vi "get_center.vi"(8 "error in (no error)":errorcluster, 11 "RoiGeneric in":refnum<class "RoiGeneric.lvclass">) -> (0 "error out":errorcluster, 2 "center":refnum<class "SpaceVector.lvclass">, 3 "RoiGeneric out":refnum<class "RoiGeneric.lvclass">)   [LabVIEW 2010, in "RoiGeneric.lvclass"]
uses:
  RoiGeneric.lvclass
  common/classes/SpaceVector/SpaceVector/SpaceVector.lvclass
  RoiGeneric.lvclass/RoiGeneric.ctl
  common/classes/Box/Box/Box.lvclass
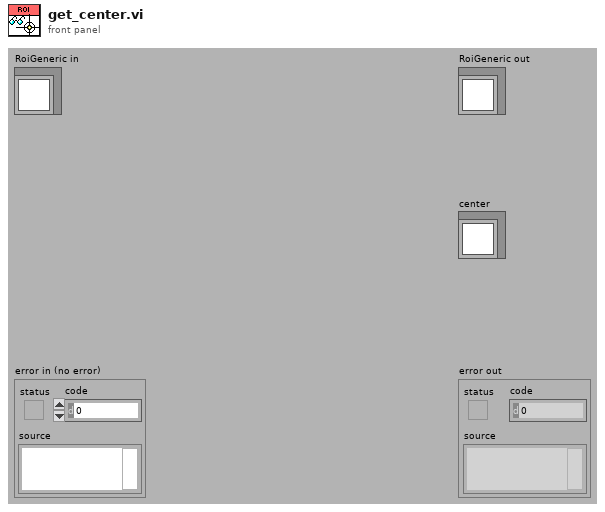
[diagram p1: front panel]
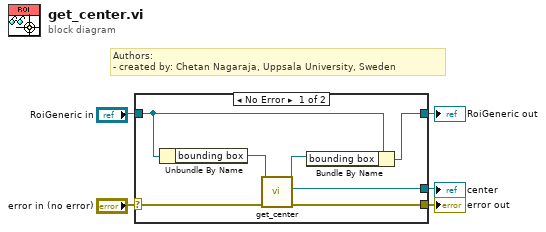
[diagram p0: block diagram]
diagram:
  # "Authors: \n- created by: Chetan Nagaraja, Uppsala University, Sweden"
  n1 = case shown="No Error" "error in (no error)" {
    selector: "error in (no error)" -> [w8 w14]
    tunnel: [w7 w14] -> w4
    tunnel: [w10 w13] -> w2
    tunnel: "RoiGeneric in" -> [w11 w13]
    tunnel: [w6 _] -> w1
    frame No Error {
      n2 = Unbundle By Name(w11) -> ("bounding box"=w12:refnum<class "Box.lvclass">)
      n3 = call "get_center.vi"("error in (no error)"=w8, "Box in"=w12) -> ("error out"=w7:errorcluster, "center"=w6:refnum<class "SpaceVector.lvclass">, "Box out"=w9:refnum<class "Box.lvclass">)  [unwired: 7 in]
      n4 = Bundle By Name(cluster=w11, "bounding box"=w9) -> (w10:refnum<class "RoiGeneric.lvclass">)
    }
    frame Error {
    }
  }
  "error out" <- w4
  "RoiGeneric out" <- w2
  "center" <- w1
